vi "_ASIC_TEST.vi"() -> ()   [LabVIEW 2009]
uses:
  global_FT Handle.vi
panel:
  out "Scaler 3 (20,21)":u16 format="%04x"
  out "Scaler 2 (18,19)":u16 format="%04x"
  out "Scaler 1 (16,17)":u16 format="%04x"
  out "Lectura asic (14,15)":u16 format="%04x"
  out "Vent. Sacaler (11,12,13)":u32 format="%06x"
  out "Periodo VGa (9,10)":u16 format="%04x"
  out "Pulse VGa (7,8)":u16 format="%04x"
  out "Ganacia VGA (6)":u8 format="%02x"
  out "adc (4,5)":u16 format="%04x"
  out "Asic (1,2,3)":u32 format="%06x"
  out "DIR 0 (CONFIG)":bool[](array[boolean])
  out "ERROR":bool
  out "UPDATE":bool
  in  "stop":bool
  out "DAC_IB":bool[](array[boolean])
  out "BUFF_ENA":bool
  out "LVDS_ENA1":bool
  out "LVDS_ENA0":bool
  out "MUX_ENA":string
  out "MUX_ENA#":i32
  out "IN 0":bool[](array[boolean])
  out "IN 6":bool[](array[boolean])
  out "IN 5":bool[](array[boolean])
  out "IN 4":bool[](array[boolean])
  out "IN 3":bool[](array[boolean])
  out "IN 2":bool[](array[boolean])
  out "IN 1":bool[](array[boolean])
  out "DAC_MUX#":i32
  out "DAC_MUX":string
  out "TH5":u16 format="%010b"
  out "TH4":u16 format="%010b"
  out "TH3":u16 format="%010b"
  out "TH2":u16 format="%010b"
  out "TH1":u16 format="%010b"
  out "TH0":u16 format="%010b"
  # "start vent. sca\nescribir ganancia\nactualizar pulso\nenable pulso\nstart tx asic\nreset asic\nescribir adc"
  # "Control_byte\nNum bit        Función\n0            \"Escribir\" ADC\n1                      \"INIT_R\" ASIC (reset)\n2                      \"start_tx\" ASIC para configuración ASIC\n3                      \"enable\" para el pulso\n4                      \"actualizar\" para el pulso\n5                      \"Escribir_ganancia\" para configuración ganancia\n6                      \"start\" para apertura ventana temportal scalers"
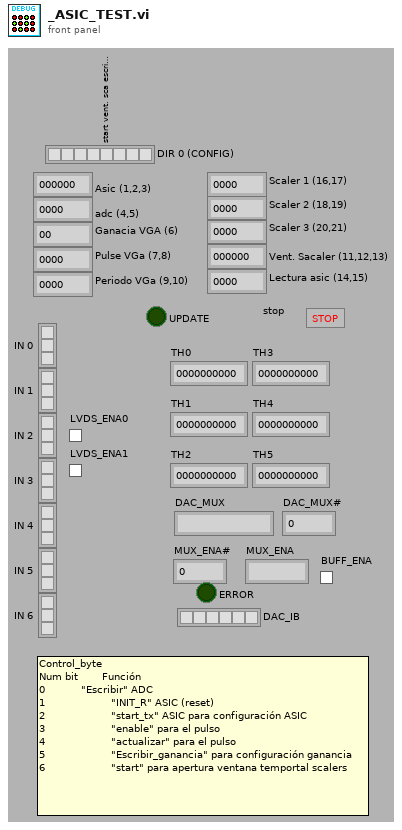
[diagram p1: front panel]
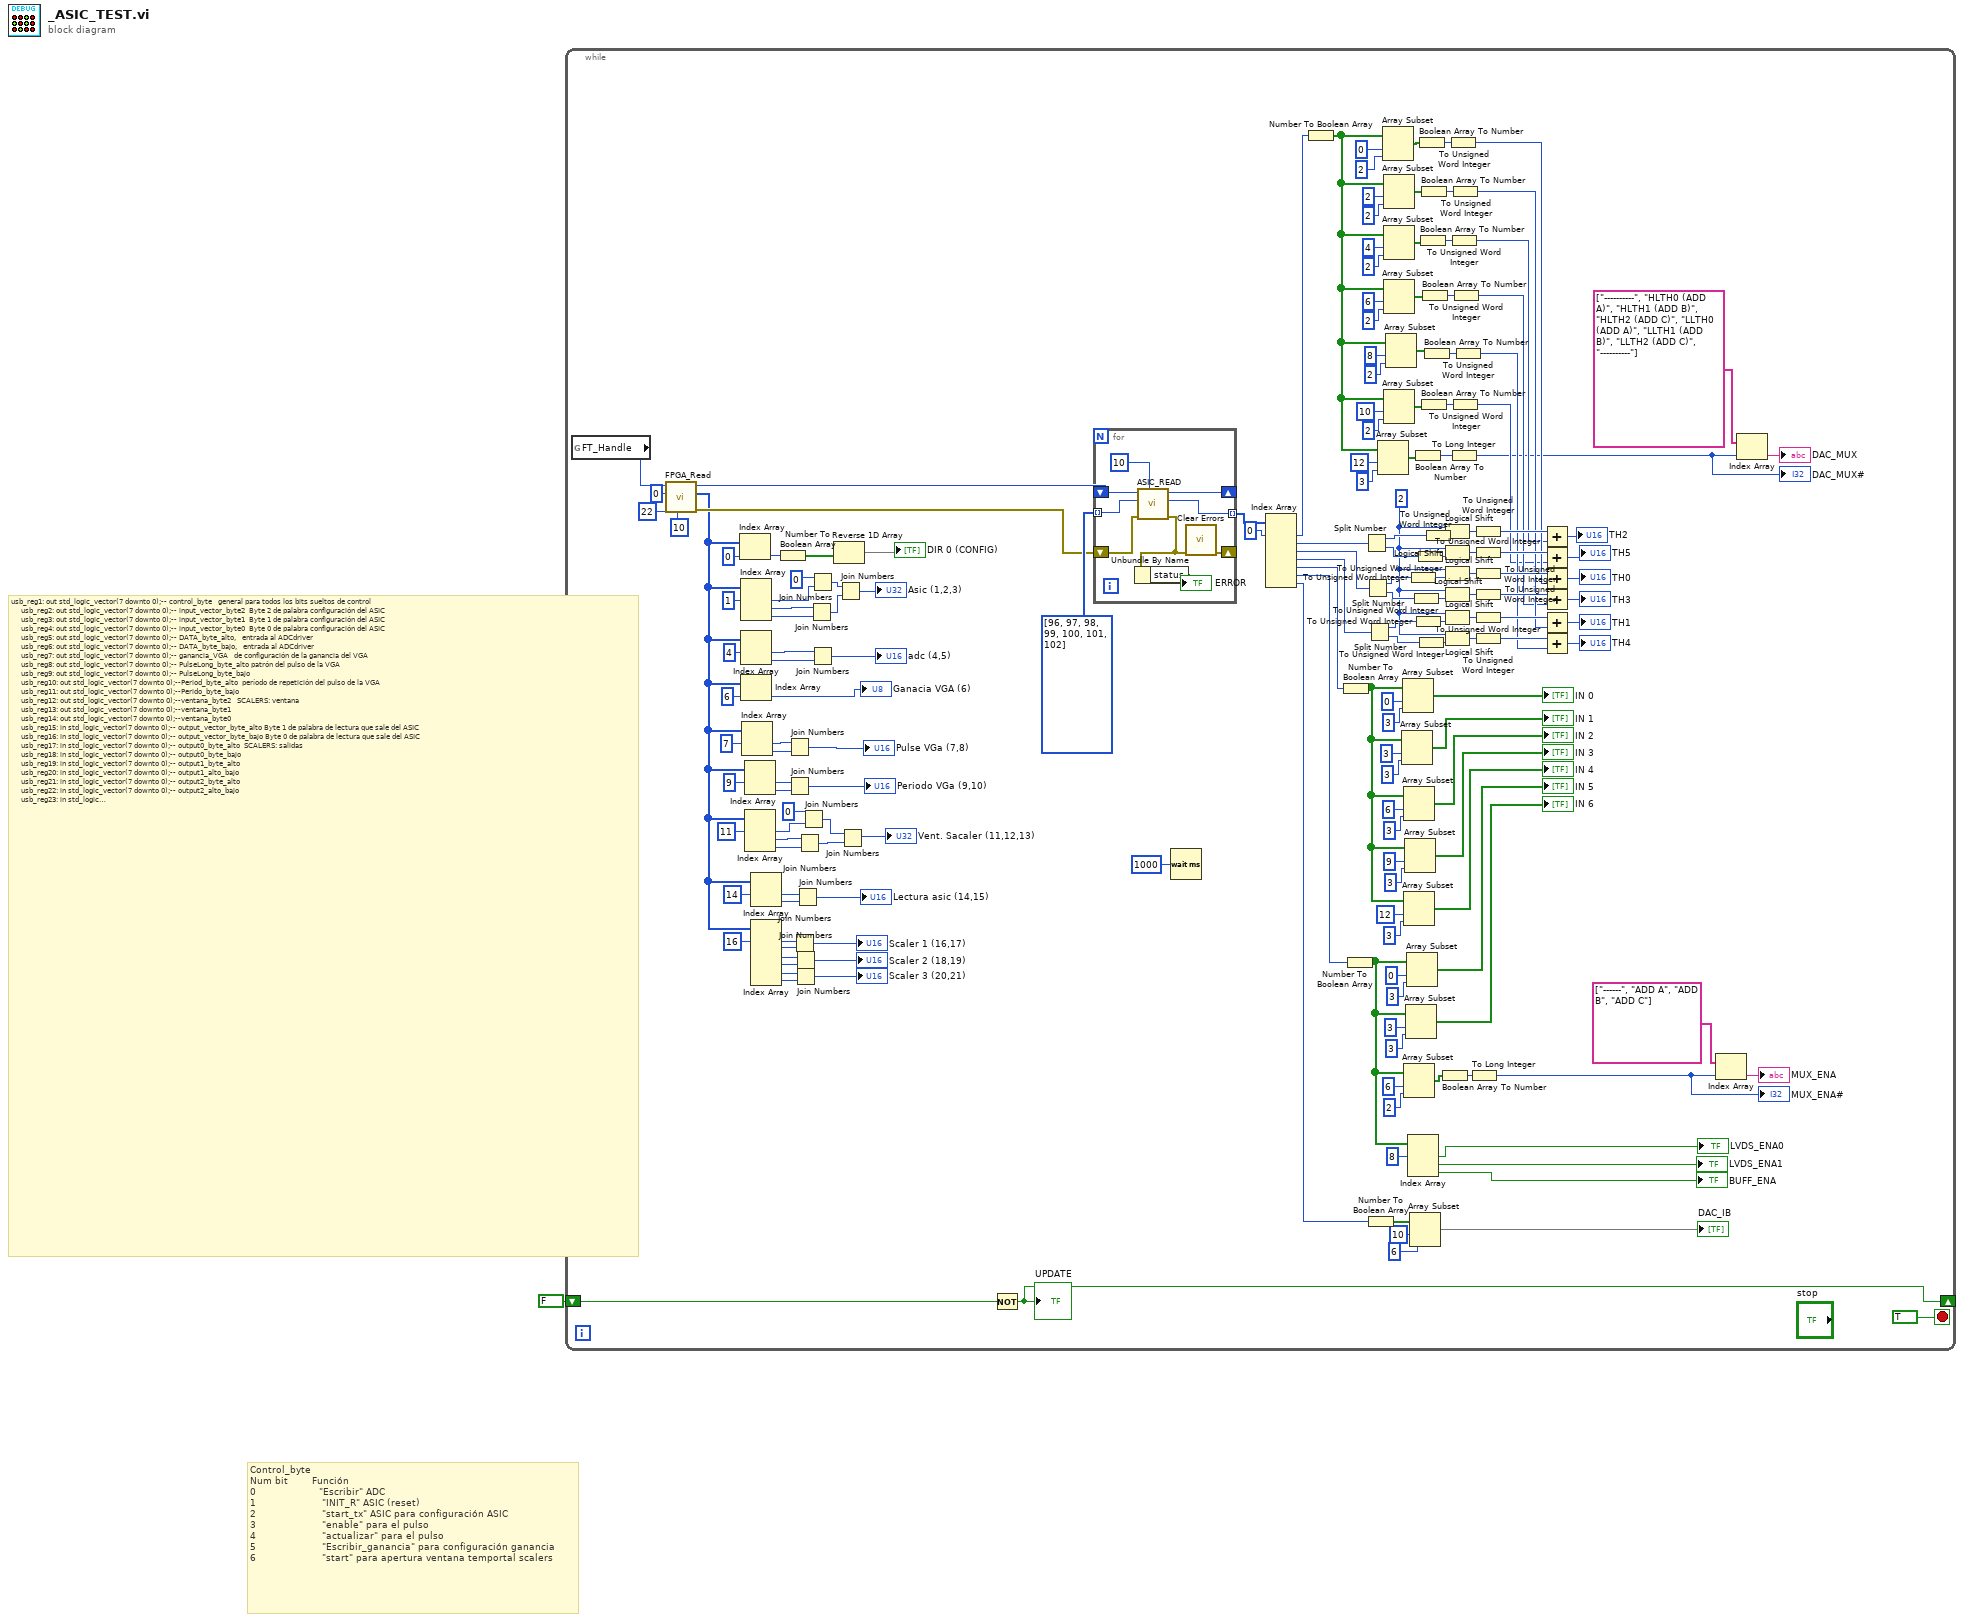
[diagram p0: block diagram]
diagram:
  # "Control_byte\nNum bit        Función\n0                     \"Escribir\" ADC\n1                      \"INIT_R\" ASIC (reset)\n2                      \"start_tx\" ASIC para configuración ASIC\n3                      \"enable\" para el pulso\n4                      \"actualizar\" para el pulso\n5                      \"Escribir_ganancia\" para configuración ganancia\n6                      \"start\" para apertura ventana temportal scalers"
  # "usb_reg1: out std_logic_vector(7 downto 0);-- control_byte\t\t\tgeneral para todos los bits sueltos de control\n\t\t\t  usb_reg2: out std_logic_vector(7 downto 0);-- input_vector_byte2 \tByte 2 de palabra configuración del ASIC\n\t\t\t  usb_reg3: out std_logic_vector(7 downto 0);-- input_vector_byte1 \tByte 1 de palabra configuración del ASIC\n\t\t\t  usb_reg4: out std_logic_vector(7 downto 0);-- input_vector_byte0 \tByte 0 de palabra configuración del ASIC\n\t\t\t  usb_reg5: out std_logic_vector(7 downto 0);-- DATA_byte_alto, \t\tentrada al ADCdriver\n\t\t\t  usb_reg6: out std_logic_vector(7 downto 0);-- DATA_byte_bajo, \t\tentrada al ADCdriver\n\t\t\t  usb_reg7: out std_logic_vector(7 downto 0);-- ganancia_VGA\t\t\tde configuración de la ganancia del VGA\n\t\t\t  usb_reg8: out std_logic_vector(7 downto 0);-- PulseLong_byte_alto\tpatrón del pulso de la VGA\n\t\t\t  usb_reg9: out std_logic_vector(7 downto 0);-- PulseLong_byte_bajo\n\t\t\t  usb_reg10: out std_logic_vector(7 downto 0);--Period_byte_alto\t\tperíodo de repetición del pulso de la VGA\n\t\t\t  usb_reg11: out std_logic_vector(7 downto 0);--Perido_byte_bajo\n\t\t\t  usb_reg12: out std_logic_vector(7 downto 0);--ventana_byte2\t\t\tSCALERS: ventana\n\t\t\t  usb_reg13: out std_logic_vector(7 downto 0);--ventana_byte1\t\n\t\t\t  usb_reg14: out std_logic_vector(7 downto 0);--ventana_byte0\n\t\t\t  usb_reg15: in std_logic_vector(7 downto 0);-- output_vector_byte_alto\tByte 1 de palabra de lectura que sale del ASIC\n\t\t\t  usb_reg16: in std_logic_vector(7 downto 0);-- output_vector_byte_bajo\tByte 0 de palabra de lectura que sale del ASIC\n\t\t\t  usb_reg17: in std_logic_vector(7 downto 0);-- output0_byte_alto\t\tSCALERS: salidas\n\t\t\t  usb_reg18: in std_logic_vector(7 downto 0);-- output0_byte_bajo\n\t\t\t  usb_reg19: in std_logic_vector(7 downto 0);-- output1_byte_alto\n\t\t\t  usb_reg20: in std_logic_vector(7 downto 0);-- output1_alto_bajo \n\t\t\t  usb_reg21: in std_logic_vector(7 downto 0);-- output2_byte_alto \n\t\t\t  usb_reg22: in std_logic_vector(7 downto 0);-- output2_alto_bajo \n\t\t\t  usb_reg23: in std_logic_vector(7 downto 0);-- para el canal_0 del ADCdriver\n\t\t\t  usb_reg24: in std_logic_vector(7 downto 0);\n\t\t\t  usb_reg25: in std_logic_vector(7 downto 0);-- para el canal_1 del ADCdriver\n\t\t\t  usb_reg26: in std_logic_vector(7 downto 0);\n\t\t\t  usb_reg27: in std_logic_vector(7 downto 0);-- para el canal_2 del ADCdriver\n\t\t\t  usb_reg28: in std_logic_vector(7 downto 0);\n\t\t\t  usb_reg29: in std_logic_vector(7 downto 0);-- para el canal_3 del ADCdriver\n\t\t\t  usb_reg30: in std_logic_vector(7 downto 0);\n\t\t\t  usb_reg31: in std_logic_vector(7 downto 0);-- para el canal_4 del ADCdriver\n\t\t\t  usb_reg32: in std_logic_vector(7 downto 0);\n\t\t\t  usb_reg33: in std_logic_vector(7 downto 0);-- para el canal_5 del ADCdriver\n\t\t\t  usb_reg34: in std_logic_vector(7 downto 0);\n\t\t\t  usb_reg35: in std_logic_vector(7 downto 0);-- para el canal_6 del ADCdriver\n\t\t\t  usb_reg36: in std_logic_vector(7 downto 0);\n\t\t\t  usb_reg37: in std_logic_vector(7 downto 0);-- para el canal_7 del ADCdriver\n\t\t\t  usb_reg38: in std_logic_vector(7 downto 0);\n\t\t\t  usb_reg39: in std_logic_vector(7 downto 0);-- para el canal_8 del ADCdriver\n\t\t\t  usb_reg40: in std_logic_vector(7 downto 0);\n\t\t\t  usb_reg41: in std_logic_vector(7 downto 0);-- para el canal_9 del ADCdriver\n\t\t\t  usb_reg42: in std_logic_vector(7 downto 0);\n\t\t\t  usb_reg43: in std_logic_vector(7 downto 0);-- para el canal_10 del ADCdriver\n\t\t\t  usb_reg44: in std_logic_vector(7 downto 0)--;"
  n1 = while {
    shift-right: [w64] -> _
    shift-left: FALSE -> [w65]
    stop <- TRUE stop-if-true
    w166 = i8 2 ("y")
    n2 = global read "global_FT Handle.vi" "FT_Handle"() -> (w57:u32)
    n3 = call "FPGA_Read.vi"("Espera acceso USB"=u32 10, "Numero Bytes"=u8 22, "Dirección base"=u8 0, "ftHandle_in"=w57) -> ("error out"=w54:errorcluster, "lpBuffer_out"=w13:u8[], "ftHandle_out"=w56:u32)  [unwired: 3 in, 2 out]
    n4 = Index Array(array=w13, index=0) -> (element=w35:u8)
    n5 = Index Array(array=w13, index #1=1 ("index")) -> (element #1=w30:u8, element #2=w31:u8, element #3=w32:u8)  [unwired: 2 in]
    n6 = Index Array(array=w13, index #1=4 ("index")) -> (element #1=w29:u8, element #2=w28:u8)  [unwired: 1 in]
    n7 = Index Array(array=w13, index=6) -> (element=→"Ganacia VGA (6)":u8)
    n8 = Index Array(array=w13, index #1=7 ("index")) -> (element #1=w22:u8, element #2=w23:u8)  [unwired: 1 in]
    n9 = Index Array(array=w13, index #1=9 ("index")) -> (element #1=w20:u8, element #2=w21:u8)  [unwired: 1 in]
    n10 = Index Array(array=w13, index #1=11 ("index")) -> (element #1=w16:u8, element #2=w14:u8, element #3=w15:u8)  [unwired: 2 in]
    n11 = Index Array(array=w13, index #1=14 ("index")) -> (element #1=w12:u8, element #2=w11:u8)  [unwired: 1 in]
    n12 = Index Array(array=w13, index #1=16 ("index")) -> (element #1=w9:u8, element #2=w8:u8, element #3=w6:u8, element #4=w5:u8, element #5=w4:u8, element #6=w3:u8)  [unwired: 5 in]
    n13 = Number To Boolean Array(number=w35) -> (Boolean array=w37:bool[])
    n14 = Join Numbers(hi=w22, lo=w23) -> ((hi.lo)=→"Pulse VGa (7,8)":u16)
    n15 = Join Numbers(hi=w20, lo=w21) -> ((hi.lo)=→"Periodo VGa (9,10)":u16)
    n16 = Join Numbers(hi=w9, lo=w8) -> ((hi.lo)=→"Scaler 1 (16,17)":u16)
    n17 = Join Numbers(hi=w6, lo=w5) -> ((hi.lo)=→"Scaler 2 (18,19)":u16)
    n18 = Join Numbers(hi=w4, lo=w3) -> ((hi.lo)=→"Scaler 3 (20,21)":u16)
    n19 = Join Numbers(hi=w12, lo=w11) -> ((hi.lo)=→"Lectura asic (14,15)":u16)
    n20 = Join Numbers(hi=w14, lo=w15) -> ((hi.lo)=w46:u16)
    n21 = Join Numbers(hi=u8 0, lo=w16) -> ((hi.lo)=w40:u16)
    n22 = Join Numbers(hi=w31, lo=w32) -> ((hi.lo)=w51:u16)
    n23 = Join Numbers(hi=u8 0, lo=w30) -> ((hi.lo)=w50:u16)
    n24 = Join Numbers(hi=w29, lo=w28) -> ((hi.lo)=→"adc (4,5)":u16)
    n25 = Reverse 1D Array(array=w37) -> (reversed array=→"DIR 0 (CONFIG)":bool[])
    n26 = Join Numbers(hi=w50, lo=w51) -> ((hi.lo)=→"Asic (1,2,3)":u32)
    n27 = Join Numbers(hi=w40, lo=w46) -> ((hi.lo)=→"Vent. Sacaler (11,12,13)":u32)
    n28 = Not(x=w65) -> (.not. x?=w64:bool)
    "UPDATE" <- w64
    n29 = for {
      tunnel: u8[] [96, 97, 98, 99, 100, 101, 102] -> [w184] mode=indexing
      tunnel: [w182] -> w176 mode=indexing
      shift-right: [w183] -> _
      shift-left: w56 -> [w186]
      shift-right: [w181] -> _
      shift-left: w54 -> [w180]
      n30 = call "ASIC_READ.vi"("Espera acceso USB"=u32 10, "error in"=w180, "Direccion Registro Asic"=w184, "ftHandle_in"=w186) -> ("error out"=w179:errorcluster, "Valor Asic"=w182:u16, "ftHandle_out"=w183:u32)  [unwired: 5 in]
      n31 = Unbundle By Name(w179) -> ("status"=→"ERROR":bool)
      n32 = call <vilib>:"Clear Errors.vi"("error in (no error)"=w179) -> ("error out"=w181:errorcluster)  [unwired: 6 in]
    }
    n33 = Wait (ms)(milliseconds to wait=u32 1000) -> ()  [unwired: 1 out]
    n34 = Index Array(array=w176, index #1=0 ("index")) -> (element #1=w108:u16, element #2=w117:u16, element #3=w174:u16, element #4=w173:u16, element #5=w107:u16, element #6=w86:u16, element #7=w70:u16)  [unwired: 6 in]
    n35 = Number To Boolean Array(number=w108) -> (Boolean array=w112:bool[])
    n36 = Number To Boolean Array(number=w107) -> (Boolean array=w95:bool[])
    n37 = Number To Boolean Array(number=w86) -> (Boolean array=w76:bool[])
    n38 = Split Number(x=w117) -> (hi(x)=w172:u8, lo(x)=w171:u8)
    n39 = Split Number(x=w174) -> (hi(x)=w170:u8, lo(x)=w169:u8)
    n40 = Split Number(x=w173) -> (hi(x)=w168:u8, lo(x)=w167:u8)
    n41 = Number To Boolean Array(number=w70) -> (Boolean array=w71:bool[])
    n42 = Array Subset(array=w112, index=12, length=3) -> (w116:bool[])
    n43 = Array Subset(array=w112, index=0, length=2) -> (w163:bool[])
    n44 = Array Subset(array=w112, index=2, length=2) -> (w144:bool[])
    n45 = Array Subset(array=w112, index=4, length=2) -> (w142:bool[])
    n46 = Array Subset(array=w112, index=6, length=2) -> (w140:bool[])
    n47 = Array Subset(array=w112, index=10, length=2) -> (w136:bool[])
    n48 = Array Subset(array=w112, index=8, length=2) -> (w138:bool[])
    n49 = Array Subset(array=w95, index=3, length=3) -> (→"IN 1":bool[])
    n50 = Array Subset(array=w95, index=0, length=3) -> (→"IN 0":bool[])
    n51 = Array Subset(array=w95, index=6, length=3) -> (→"IN 2":bool[])
    n52 = Array Subset(array=w95, index=12, length=3) -> (→"IN 4":bool[])
    n53 = Array Subset(array=w76, index=6, length=2) -> (w79:bool[])
    n54 = Array Subset(array=w95, index=9, length=3) -> (→"IN 3":bool[])
    n55 = Array Subset(array=w76, index=3, length=3) -> (→"IN 6":bool[])
    n56 = Array Subset(array=w76, index=0, length=3) -> (→"IN 5":bool[])
    n57 = To Unsigned Word Integer(number=w170) -> (unsigned 16bit integer=w60:u16)
    n58 = Index Array(array=w76, index #1=8 ("index")) -> (element #1=→"LVDS_ENA0":bool, element #2=→"LVDS_ENA1":bool, element #3=→"BUFF_ENA":bool)  [unwired: 2 in]
    n59 = Array Subset(array=w71, index=10, length=6) -> (→"DAC_IB":bool[])
    n60 = To Unsigned Word Integer(number=w169) -> (unsigned 16bit integer=w61:u16)
    n61 = Boolean Array To Number(Boolean array=w116) -> (number=w115:u32)
    n62 = To Unsigned Word Integer(number=w168) -> (unsigned 16bit integer=w62:u16)
    n63 = To Unsigned Word Integer(number=w171) -> (unsigned 16bit integer=w59:u16)
    n64 = To Unsigned Word Integer(number=w167) -> (unsigned 16bit integer=w63:u16)
    n65 = Boolean Array To Number(Boolean array=w163) -> (number=w161:u32)
    n66 = Boolean Array To Number(Boolean array=w142) -> (number=w143:u32)
    n67 = Boolean Array To Number(Boolean array=w144) -> (number=w145:u32)
    n68 = Boolean Array To Number(Boolean array=w136) -> (number=w137:u32)
    n69 = Boolean Array To Number(Boolean array=w140) -> (number=w141:u32)
    n70 = Boolean Array To Number(Boolean array=w138) -> (number=w139:u32)
    n71 = To Unsigned Word Integer(number=w172) -> (unsigned 16bit integer=w58:u16)
    n72 = Boolean Array To Number(Boolean array=w79) -> (number=w78:u32)
    n73 = Logical Shift(y=w166, x=w58) -> (x << y=w162:u16)
    n74 = Logical Shift(y=w166, x=w59) -> (x << y=w159:u16)
    n75 = Logical Shift(y=w166, x=w60) -> (x << y=w135:u16)
    n76 = Logical Shift(y=w166, x=w61) -> (x << y=w134:u16)
    n77 = Logical Shift(y=w166, x=w62) -> (x << y=w133:u16)
    n78 = Logical Shift(y=w166, x=w63) -> (x << y=w132:u16)
    n79 = To Unsigned Word Integer(number=w161) -> (unsigned 16bit integer=w123:u16)
    n80 = To Unsigned Word Integer(number=w143) -> (unsigned 16bit integer=w121:u16)
    n81 = To Long Integer(number=w115) -> (32bit integer=w110:i32)
    "DAC_MUX#" <- w110
    n82 = To Unsigned Word Integer(number=w145) -> (unsigned 16bit integer=w122:u16)
    n83 = To Unsigned Word Integer(number=w137) -> (unsigned 16bit integer=w118:u16)
    n84 = To Unsigned Word Integer(number=w141) -> (unsigned 16bit integer=w120:u16)
    n85 = To Unsigned Word Integer(number=w139) -> (unsigned 16bit integer=w119:u16)
    n86 = To Long Integer(number=w78) -> (32bit integer=w77:i32)
    "MUX_ENA#" <- w77
    n87 = To Unsigned Word Integer(number=w162) -> (unsigned 16bit integer=w160:u16)
    n88 = To Unsigned Word Integer(number=w159) -> (unsigned 16bit integer=w158:u16)
    n89 = To Unsigned Word Integer(number=w135) -> (unsigned 16bit integer=w131:u16)
    n90 = To Unsigned Word Integer(number=w134) -> (unsigned 16bit integer=w130:u16)
    n91 = To Unsigned Word Integer(number=w133) -> (unsigned 16bit integer=w129:u16)
    n92 = To Unsigned Word Integer(number=w132) -> (unsigned 16bit integer=w128:u16)
    n93 = Add(x=w160, y=w121) -> (x+y=→"TH2":u16)
    n94 = Add(x=w158, y=w118) -> (x+y=→"TH5":u16)
    n95 = Add(x=w131, y=w123) -> (x+y=→"TH0":u16)
    n96 = Add(x=w130, y=w120) -> (x+y=→"TH3":u16)
    n97 = Add(x=w129, y=w122) -> (x+y=→"TH1":u16)
    n98 = Add(x=w128, y=w119) -> (x+y=→"TH4":u16)
    n99 = Index Array(array=string[] ["------", "ADD A", "ADD B", "ADD C"], index=w77) -> (element=→"MUX_ENA":string)
    n100 = Index Array(array=string[] ["----------", "HLTH0 (ADD A)", "HLTH1 (ADD B)", "HLTH2 (ADD C)", "LLTH0 (ADD A)", "LLTH1 (ADD B)", "LLTH2 (ADD C)", "----------"], index=w110) -> (element=→"DAC_MUX":string)
  }
